vi "niDTS WLAN VHT Rx Test UTIL VHT Parameters to WLAN Rx Parameters.vi"(7 "WLAN Rx Input Parameters":T1={"MCS Index"=0, "N Spatial Streams"=0, "Chains"=[TRUE, FALSE, FALSE, FALSE], "Bandwidth (Hz)"=enum."160 MHz", "Channel"=0, "Power (dBm)"=0.0, "Guard Interval"=enum."SHORT", "FEC Coding"=enum."BCC", "16 symbols"=TRUE, "Payload Length (bytes)"=1500, "Idle Interval (s)"=1.0, "External Attenuation (dB)"=[0.0, 0.0, 0.0, 0.0], "RX Measurement Parameters"={"Number of Packets"=1000, "MacAddress"="FF:FF:FF:FF:FF:FF"}} {"Idle Interval (s)" format="%_3p"}) -> (8 "WLAN Tx Parameters":T6={"Standard"=enum."802.11 n HT", "DSSS Data Rate (Mbps)"=enum."1", "OFDM Data Rate (Mbps)"=enum."54", "MCS Index"=7, "N Spatial Streams"=1, "Chains"=[TRUE, FALSE, FALSE, FALSE], "Bandwidth (Hz)"=enum."20 MHz", "Channel"=1, "Power (dBm)"=0.0, "Guard Interval"=enum."SHORT", "FEC Coding"=enum."LDPC", "16 symbols"=TRUE, "Payload Length (bytes)"=1500, "Idle Interval (s)"=0.0001, "External Attenuation (dB)"=[0.0, 0.0, 0.0, 0.0], "RX Measurement Parameters"={"Number of Packets"=1000, "MacAddress"="FF:FF:FF:FF:FF:FF"}} {"Idle Interval (s)" format="%_3p"})   [LabVIEW 2014, in "niDTS WLAN.lvlib"]
uses:
  niDTS WLAN.lvlib
  Rx Test/Includes/niDTS WLAN Rx Test INC Parameters.ctl
  Includes/niDTS WLAN INC Standard.ctl
  Includes/niDTS WLAN INC DSSS Data Rate.ctl
  Includes/niDTS WLAN INC OFDM Data Rate.ctl
  Includes/niDTS WLAN INC CH BW.ctl
  Includes/niDTS WLAN INC GI.ctl
  Includes/niDTS WLAN INC FEC Coding.ctl
  Rx Test/Includes/niDTS WLAN INC RX Measurement Parameters.ctl
  Includes/niDTS WLAN VHT Rx Test INC Parameters.ctl
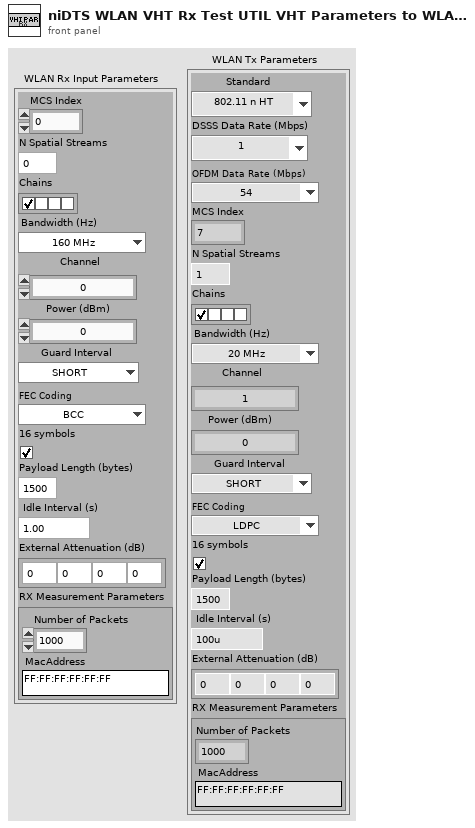
[diagram p1: front panel]
types:
  T1 = typedef "niDTS WLAN.lvlib/niDTS WLAN VHT Rx Test INC Parameters.ctl" = cluster{"MCS Index":i32, "N Spatial Streams":i32, "Chains":bool[], "Bandwidth (Hz)":T2, "Channel":i32, "Power (dBm)":dbl, "Guard Interval":T3, "FEC Coding":T4, "16 symbols":bool, "Payload Length (bytes)":i32, "Idle Interval (s)":dbl, "External Attenuation (dB)":dbl[], "RX Measurement Parameters":T5}
  T2 = typedef "niDTS WLAN.lvlib/niDTS WLAN INC CH BW.ctl" = enum16{"20 MHz", "40 MHz", "80 MHz", "160 MHz"}
  T3 = typedef "niDTS WLAN.lvlib/niDTS WLAN INC GI.ctl" = enum16{"LONG", "SHORT"}
  T4 = typedef "niDTS WLAN.lvlib/niDTS WLAN INC FEC Coding.ctl" = enum16{"BCC", "LDPC"}
  T5 = typedef "niDTS WLAN.lvlib/niDTS WLAN INC RX Measurement Parameters.ctl" = cluster{"Number of Packets":i32, "MacAddress":string}
  T6 = typedef "niDTS WLAN.lvlib/niDTS WLAN Rx Test INC Parameters.ctl" = cluster{"Standard":T7, "DSSS Data Rate (Mbps)":T8, "OFDM Data Rate (Mbps)":T9, "MCS Index":i32, "N Spatial Streams":i32, "Chains":bool[], "Bandwidth (Hz)":T2, "Channel":i32, "Power (dBm)":dbl, "Guard Interval":T3, "FEC Coding":T4, "16 symbols":bool, "Payload Length (bytes)":i32, "Idle Interval (s)":dbl, "External Attenuation (dB)":dbl[], "RX Measurement Parameters":T5}
  T7 = typedef "niDTS WLAN.lvlib/niDTS WLAN INC Standard.ctl" = enum16{"802.11 b DSSS", "802.11 a/g OFDM", "802.11 n HT", "802.11 ac VHT"}
  T8 = typedef "niDTS WLAN.lvlib/niDTS WLAN INC DSSS Data Rate.ctl" = enum16{"1", "2", "5.5", "11"}
  T9 = typedef "niDTS WLAN.lvlib/niDTS WLAN INC OFDM Data Rate.ctl" = enum16{"6", "9", "12", "18", "24", "36", "48", "54"}
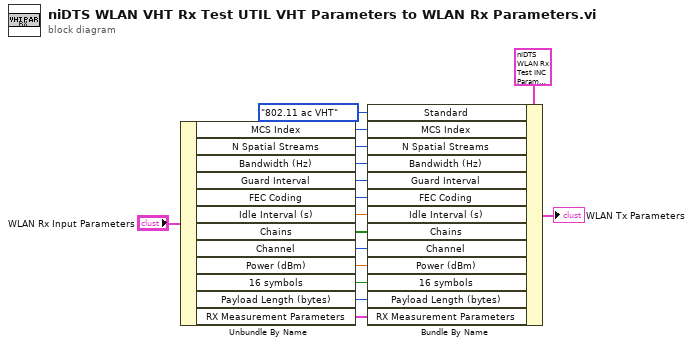
[diagram p0: block diagram]
diagram:
  n1 = Unbundle By Name("WLAN Rx Input Parameters") -> ("MCS Index"=w16:i32, "N Spatial Streams"=w15:i32, "Bandwidth (Hz)"=w14:T2, "Guard Interval"=w13:T3, "FEC Coding"=w12:T4, "Idle Interval (s)"=w11:dbl, "Chains"=w10:bool[], "Channel"=w9:i32, "Power (dBm)"=w8:dbl, "16 symbols"=w7:bool, "Payload Length (bytes)"=w6:i32, "RX Measurement Parameters"=w5:T5)
  n2 = Bundle By Name(cluster=T6 {"Standard"=enum."802.11 n HT", "DSSS Data Rate (Mbps)"=enum."1", "OFDM Data Rate (Mbps)"=enum."54", "MCS Index"=7, "N Spatial Streams"=1, "Chains"=[TRUE, FALSE, FALSE, FALSE], "Bandwidth (Hz)"=enum."20 MHz", "Channel"=1, "Power (dBm)"=0.0, "Guard Interval"=enum."SHORT", "FEC Coding"=enum."LDPC", "16 symbols"=TRUE, "Payload Length (bytes)"=1500, "Idle Interval (s)"=0.0001, "External Attenuation (dB)"=[0.0, 0.0, 0.0, 0.0], "RX Measurement Parameters"={"Number of Packets"=1000, "MacAddress"="FF:FF:FF:FF:FF:FF"}} ("WLAN Rx Input Parameters"), "Standard"=niDTS_WLAN_INC_Standard."802.11 ac VHT", "MCS Index"=w16, "N Spatial Streams"=w15, "Bandwidth (Hz)"=w14, "Guard Interval"=w13, "FEC Coding"=w12, "Idle Interval (s)"=w11, "Chains"=w10, "Channel"=w9, "Power (dBm)"=w8, "16 symbols"=w7, "Payload Length (bytes)"=w6, "RX Measurement Parameters"=w5) -> (→"WLAN Tx Parameters":T6)
